vi "testfiles.vi"() -> ()   [LabVIEW 2011]
uses:
  <vilib>/vision/NI_Vision_Development_Module.lvlib
panel:
  out "same":bool
  out "appended path 2":path=path "V:/Test/Y2013/04-Apr/13_0426/scans/Scan002/MagCam3/Scan002_StagingMagSpec_042_Cam3.png"
  out "appended path":path=path "V:/Test/Y2013/04-Apr/13_0426/scans/Scan002/MagCam3/Scan002_StagingMagSpec_043_Cam3.png"
  out "Array":bool[](array[boolean])
  in  "File Path 3":path=path "V:/Test/Y2013/04-Apr/13_0426/scans/Scan002/MagCam3"
  out "Histogram Report":T1={"histogram"=[0, 0, 0, 41799, 0, 0, 0, 0, 0, 9230, 0, 0, 0, 0, 0, 8883, 0, 0, 0, 0, 0, 8253, 0, 0, 0, 0, 0, 0, 7232, 0, 0, 0, 0, 0, 6124, 0, 0, 0, 0, 0, 5141, 0, 0, 0, 0, 0, 4093, 0, 0, 0, 0, 0, 0, 3173, 0, 0, 0, 0, 0, 2430, 0, 0, 0, 0, 0, 1979, 0, 0, 0, 0, 0, 1431, 0, 0, 0, 0, 0, 0, 1041, 0, 0, 0, 0, 0, 802, 0, 0, 0, 0, 0, 628, 0, 0, 0, 0, 0, 427, 0, 0, 0, 0, 0, 0, 326, 0, 0, 0, 0, 0, 244, 0, 0, 0, 0, 0, 176, 0, 0, 0, 0, 0, 130, 0, 0, 0, 0, 0, 81, 0, 0, 0, 0, 0, 0, 55, 0, 0, 0, 0, 0, 32, 0, 0, 0, 0, 0, 25, 0, 0, 0, 0, 0, 25, 0, 0, 0, 0, 0, 0, 11, 0, 0, 0, 0, 0, 13, 0, 0, 0, 0, 0, 6, 0, 0, 0, 0, 0, 4, 0, 0, 0, 0, 0, 0, 2, 0, 0, 0, 0, 0, 1, 0, 0, 0, 0, 0, 2, 0, 0, 0, 0, 0, 0, 0, 0, 0, 0, 0, 0, 0, 0, 0, 0, 0, 0, 0, 0, 0, 0, 0, 0, 0, 0, 0, 0, 0, 0, 0, 0, 0, 0, 0, 0, 0, 0, 0, 0, 0, 0, 0, 0, 0, 0, 0, 0, 0, 0, 0, 0, 0, 0, 0, 1, 0, 0, 0], "Minimal Value"=0.0, "Maximal Value"=40.0, "Starting Value"=0.0, "Interval Width"=0.16015625, "Mean Value"=3.0099518, "Standard  Variation"=3.795856, "Area (pixels)"=103800} {"Standard  Variation" format="%.2f"; "Mean Value" format="%.2f"; "Interval Width" format="%.2f"; "Starting Value" format="%.2f"; "Maximal Value" format="%.2f"; "Minimal Value" format="%.2f"}
  out "Image":T2(plugin-control)
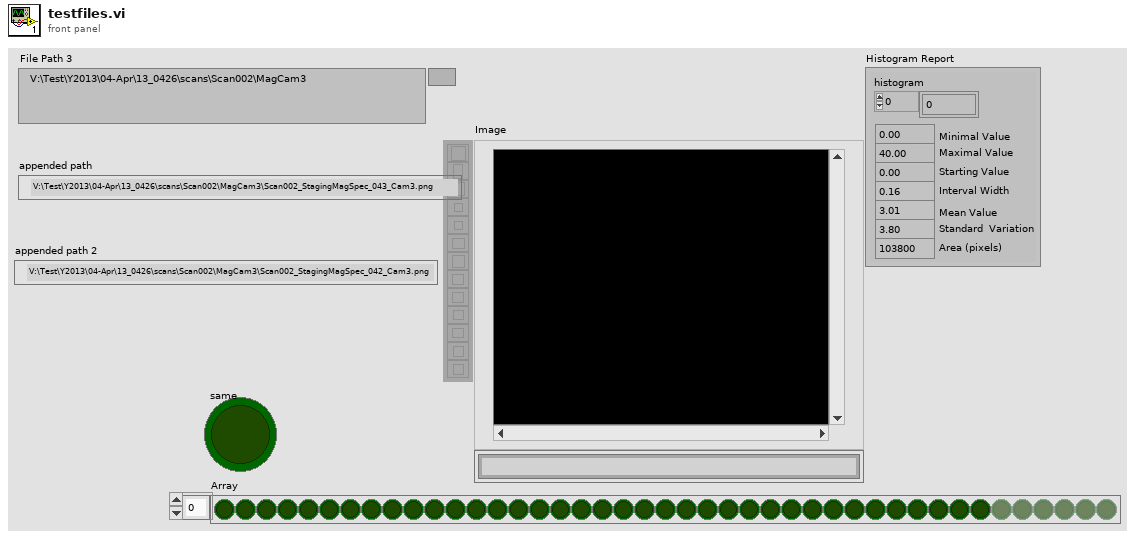
[diagram p1: front panel]
types:
  T1 = cluster{"histogram":u32[], "Minimal Value":sgl, "Maximal Value":sgl, "Starting Value":sgl, "Interval Width":sgl, "Mean Value":sgl, "Standard  Variation":sgl, "Area (pixels)":i32}
  T2 = typedef "IMAQ Image.ctl" = refnum<image>
  T3 = typedef "Image Type" = u32
  T4 = enum32{"Average", "Min", "Max", "Clear  if < ", "Clear  if < or =", "Clear  if =", "Clear  if > or =", "Clear  if >"}
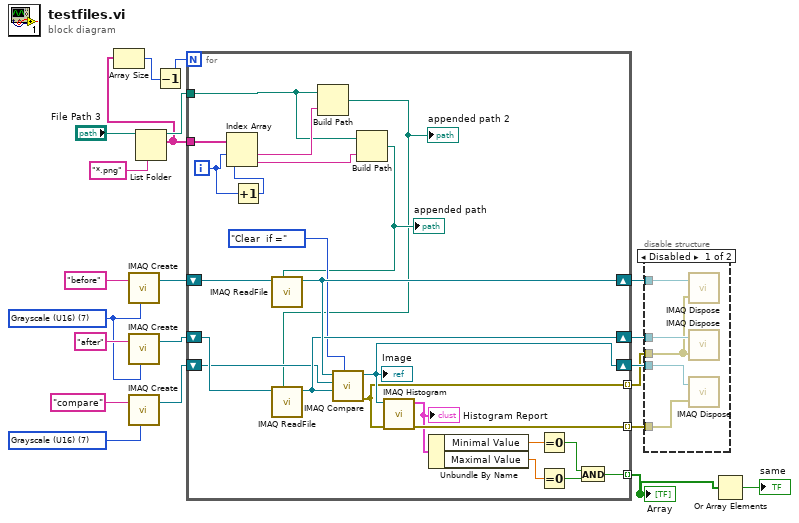
[diagram p0: block diagram]
diagram:
  w14 = T3 7 items=["Grayscale (U8)", "Grayscale (I16)", "Grayscale (SGL)", "Complex (CSG)", "RGB (U32)", "HSL (U32)", "RGB (U64)", "Grayscale (U16)"] ("Image Type")
  w19 = T3 7 items=["Grayscale (U8)", "Grayscale (I16)", "Grayscale (SGL)", "Complex (CSG)", "RGB (U32)", "HSL (U32)", "RGB (U64)", "Grayscale (U16)"] ("Image Type")
  n1 = call "IMAQ Create"("Image Name"="before", "Image Type"=w19) -> ("New Image"=w18:T2)  [unwired: 3 in, 1 out]
  n2 = call "IMAQ Create"("Image Name"="after", "Image Type"=w19) -> ("New Image"=w17:T2)  [unwired: 3 in, 1 out]
  n3 = call "IMAQ Create"("Image Name"="compare", "Image Type"=w14) -> ("New Image"=w12:T2)  [unwired: 3 in, 1 out]
  n4 = List Folder(path="File Path 3", pattern="*.png") -> (path out=w7:path, filenames=w6:string[])  [unwired: 2 in, 2 out]
  n5 = Array Size(array=w6) -> (size(s)=w5:i32)
  n6 = Decrement(x=w5) -> (x-1=w4:i32)
  n7 = for {
    N: w4 -> [_]
    tunnel: [w37] -> w10 mode=indexing
    tunnel: [w36] -> w9 mode=indexing
    tunnel: [w30] -> w2 mode=indexing
    shift-right: [w42] -> w16
    shift-left: w18 -> [w44]
    shift-right: [w38] -> w11
    shift-left: w12 -> [w39]
    shift-right: [w41] -> w15
    shift-left: w17 -> [w43]
    tunnel: w6 -> [w29]
    tunnel: w7 -> [w26]
    i -> [w23]
    n8 = Increment(x=w23) -> (x+1=w22:i32)
    n9 = Index Array(array=w29, index #1=w23, index #2=w22) -> (element #1=w28:string, element #2=w27:string)
    n10 = Build Path(base path=w26, name or relative path=w28) -> (appended path=w24:path)
    "appended path 2" <- w24
    n11 = call "IMAQ ReadFile"("File Path"=w24, "Image"=w43) -> ("Image Out"=w41:T2)  [unwired: 5 in, 4 out]
    n12 = Build Path(base path=w26, name or relative path=w27) -> (appended path=w25:path)
    "appended path" <- w25
    n13 = call "IMAQ ReadFile"("File Path"=w25, "Image"=w44) -> ("Image Out"=w42:T2)  [unwired: 5 in, 4 out]
    n14 = call "IMAQ Compare"("Operator"=T4."Clear  if =", "Image Src B"=w41, "Image Dst"=w39, "Image Src A"=w42) -> ("error out"=w37:errorcluster, "Image Dst Out"=w38:T2)  [unwired: 6 in]
    "Image" <- w38
    n15 = call "IMAQ Histogram"("error in (no error)"=w37, "Image"=w38) -> ("error out"=w36:errorcluster, "Histogram Report"=w35:T1)  [unwired: 8 in]
    "Histogram Report" <- w35
    n16 = Unbundle By Name(w35) -> ("Minimal Value"=w34:sgl, "Maximal Value"=w33:sgl)
    n17 = Equal To 0?(x=w34) -> (x = 0?=w32:bool)
    n18 = Equal To 0?(x=w33) -> (x = 0?=w31:bool)
    n19 = And(x=w32, y=w31) -> (x .and. y?=w30:bool)
  }
  "Array" <- w2
  n20 = disable-structure shown="Disabled" {
    disable-tunnel: w16 -> [w49 _]
    disable-tunnel: w15 -> [w48 _]
    disable-tunnel: w11 -> [w47 _]
    disable-tunnel: w10 -> [w46 _]
    disable-tunnel: w9 -> [w45 _]
    frame Disabled {
      n21 = call "IMAQ Dispose"("Image"=w49, "error in (no error)"=w46) -> ()  [unwired: 4 in, 1 out]
      n22 = call "IMAQ Dispose"("Image"=w48, "error in (no error)"=w46) -> ()  [unwired: 4 in, 1 out]
      n23 = call "IMAQ Dispose"("Image"=w47, "error in (no error)"=w45) -> ()  [unwired: 4 in, 1 out]
    }
    frame Enabled {
    }
  }
  n24 = Or Array Elements(Boolean array=w2) -> (logical OR=→"same":bool)
